vi "CreateIntegerArrayJ&J.vi"(10 "Cluster":T1) -> (2 "Array":dbl[](array[numeric]))   [LabVIEW 2015]
uses:
  <vilib>/imath/engines/lvmath2/RunTimeEngine/Managers/WorkSpace/UID Generator.vi
  <vilib>/imath/engines/lvmath2/RunTimeEngine/RunTimeType/NIMS_RunTimeType_From StrictType (excl LVString).vi
  <instcachedir>/0/NIMS_RunTimeType_From StrictType (excl LVString)_EB1C38A9BC5048DA9ABDA8F781E54D21.lvgen/NIMS_RunTimeType_From StrictType (excl LVString)_EB1C38A9BC5048DA9ABDA8F781E54D21_000.vi
  <vilib>/imath/engines/lvmath2/RunTimeEngine/LocalVariableDefStatement/MC_LocalVariableDefStatement_Display.vi
  <vilib>/imath/engines/lvmath2/RunTimeSupport/NIMS_Complex To Real.vi
  <instcachedir>/0/NIMS_Complex To Real_01315F44AA8B4CE79FEF95AE999DC25E.lvgen/NIMS_Complex To Real_01315F44AA8B4CE79FEF95AE999DC25E_001.vi
  <vilib>/imath/engines/lvmath2/RunTimeEngine/BuiltInFunctions/logramp/NIMS_logramp.vi
  <vilib>/imath/engines/lvmath2/RunTimeEngine/BuiltInFunctions/round/NIMS_round(DBL-V).vi
  <vilib>/imath/engines/lvmath2/RunTimeEngine/ErrorHandling/NIMS_Create Error From Enums.vi
  <vilib>/imath/engines/lvmath2/RunTimeEngine/RangeToken/NIMS_Range.vi
  <instcachedir>/0/NIMS_Range_D919CC09935940E88F755EC1C6F49AC1.lvgen/NIMS_Range_D919CC09935940E88F755EC1C6F49AC1_000.vi
  <vilib>/imathl/engines/lvmath/Functions/Error Handling/Create Error.vi
  <vilib>/imath/engines/lvmath2/RunTimeEngine/VariableToken/NIMS_VariableToken_CondDefined.vi
  <instcachedir>/0/NIMS_VariableToken_CondDefined_FE30D0A1BFB24F098D41DEBABFE96BE1.lvgen/NIMS_VariableToken_CondDefined_FE30D0A1BFB24F098D41DEBABFE96BE1_003.vi
  <vilib>/imath/engines/lvmath2/RunTimeEngine/Managers/SymbolTable/Clear UID.vi
  <vilib>/imath/engines/lvmath2/RunTimeEngine/NodeEndStatement/NIMS_NodeEndStatement_Output.vi
  <instcachedir>/0/NIMS_NodeEndStatement_Output_53EC0D466D134D7ABD903AC30B43404B.lvgen/NIMS_NodeEndStatement_Output_53EC0D466D134D7ABD903AC30B43404B_005.vi
  <vilib>/imath/engines/lvmath2/RunTimeEngine/ErrorHandling/NIMS_Finalize Error.vi
  <vilib>/imath/engines/lvmath2/RunTimeEngine/Managers/SymbolTable/NIMS_WorkSpace.lvlib
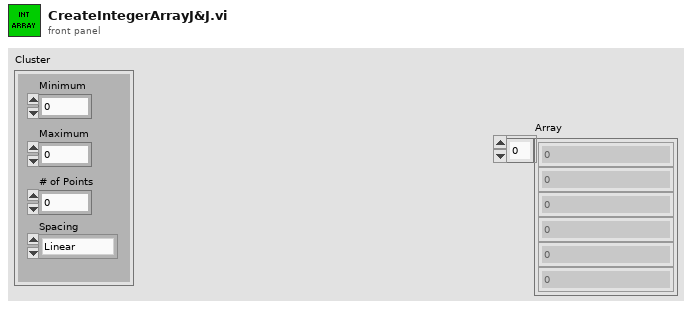
[diagram p1: front panel]
types:
  T1 = cluster{"Minimum":dbl, "Maximum":dbl, "# of Points":dbl, "Spacing":enum16{"Linear", "Logarithmic"}}
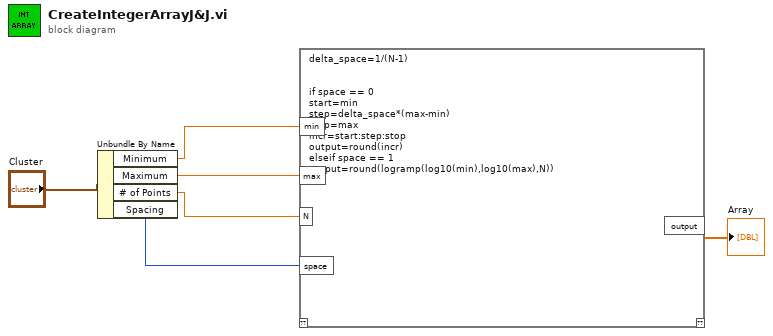
[diagram p0: block diagram]
diagram:
  n1 = Unbundle By Name("Cluster") -> ("Minimum"=w4:dbl, "Maximum"=w3:dbl, "# of Points"=w2:dbl, "Spacing"=w1:enum16{"Linear", "Logarithmic"})
  n2 = mathscript code="delta_space=1/(N-1)\n\n\nif space == 0\nstart=min\nstep=delta_space*(max-min)\nstop=max\nincr=start:step:stop\noutput=round(incr)\nelseif space == 1\noutput=round(logramp(log10(min),log10(max),N))\nend"("min"=w4, "max"=w3, "N"=w2, "space"=w1) -> ("output"=→"Array":dbl[])  [unwired: 1 in, 1 out]
